vi "IV.vi"(2 "Run uninterrupted?":bool, 3 "Device Category:":string(combo)="Short Strip", 4 "Batch No.:":string, 5 "Wafer Serial No.:":string, 6 "Sensor Serial No.:":string) -> (0 "Done!":bool)   [LabVIEW 2013]
doc: "Performs IV measurements according to ATLAS ITk Quality Control Specifications."
uses:
  InstrControl/Switching/Switching.lvclass
  InstrControl/SupplyControl/SupplyControl.lvclass
  general_VIs/globals/MeasurementSetup.vi
  general_VIs/globals/RunInformation.vi
  InstrControl/InstrumentSetup.vi
  InstrControl/ArduinoControl/ArduinoControl.lvclass
  <vilib>/Analysis/NI_AALBase.lvlib
  InstrControl/InstrControl.lvclass
panel:
  out "Initial volts [V]":dbl format="%.1f"
  out "Final volts [V]":dbl=-700.0 format="%.1f"
  out "step [V]":dbl=10.0 format="%.1f"
  out "step interval [s]":u32=10
  out "Volts":dbl[](array[numeric]) caption="Volts [V]"
  out "Current":dbl[](array[numeric]) caption="Current [nA]"
  out "Temp.":dbl[](array[numeric]) caption="Temp. [°C]" format="%#.2f"
  out "RH":dbl[](array[numeric]) caption="RH [%]" format="%#.2f"
  out "Igraph":cluster{"Initial volts":dbl, dbl, dbl[]}(graph)
  in  "Scales":T1(ring)
  in  "Iscale":enum16{"nanoAmps", "microAmps", "milliAmps"}(ring)
  out "positive ramp?":bool
  out "Tab Control":enum32{"IV Setup", "IV Scan"}(tab)
  in  "User:":string(combo)="Christoph"
  out "IV Supply":string
  in  "Configurations":bool
  in  "Set current limit?":bool
  in  "Current Limit [µA]":dbl=1000.0 min=0.0001 format="%.3f"
  in  "Manufacturer:":string(combo)="Hamamatsu"
  in  "Quit":bool
  in  "Continue":bool
  out "Temperature":enum16{"Read Arduino", "Enter manually"}(ring)
  in  "abort":bool
  out "Device Category:":string
  out "Batch:":string
  out "Current Volts:":dbl format="%.2f"
  in  "quit (no save)":bool
  in  "Quit & Save":bool
  out "Bias On/Off:":bool
  out "STATUS 1":string
  out "Initiated:":string
  out "Sensor No.:":string
  out "No of steps":u32
  out "Current reading No.":u32
  out "Last reading at:":string
  # "University of\nCambridge"
  # "Strip Sensor QC: IV"
  # "IV Scan parameters:"
  # "Last 5 readings:"
  # "n-4"
  # "n-3"
  # "n-2"
  # "n-1"
  # "n"
  # "Vertical Scale:"
  # "DUT & Test Description"
  # "Hardware"
  # "DUT & Test Description:"
  # "Current status:"
  # "Rdg No:"
  # "out of"
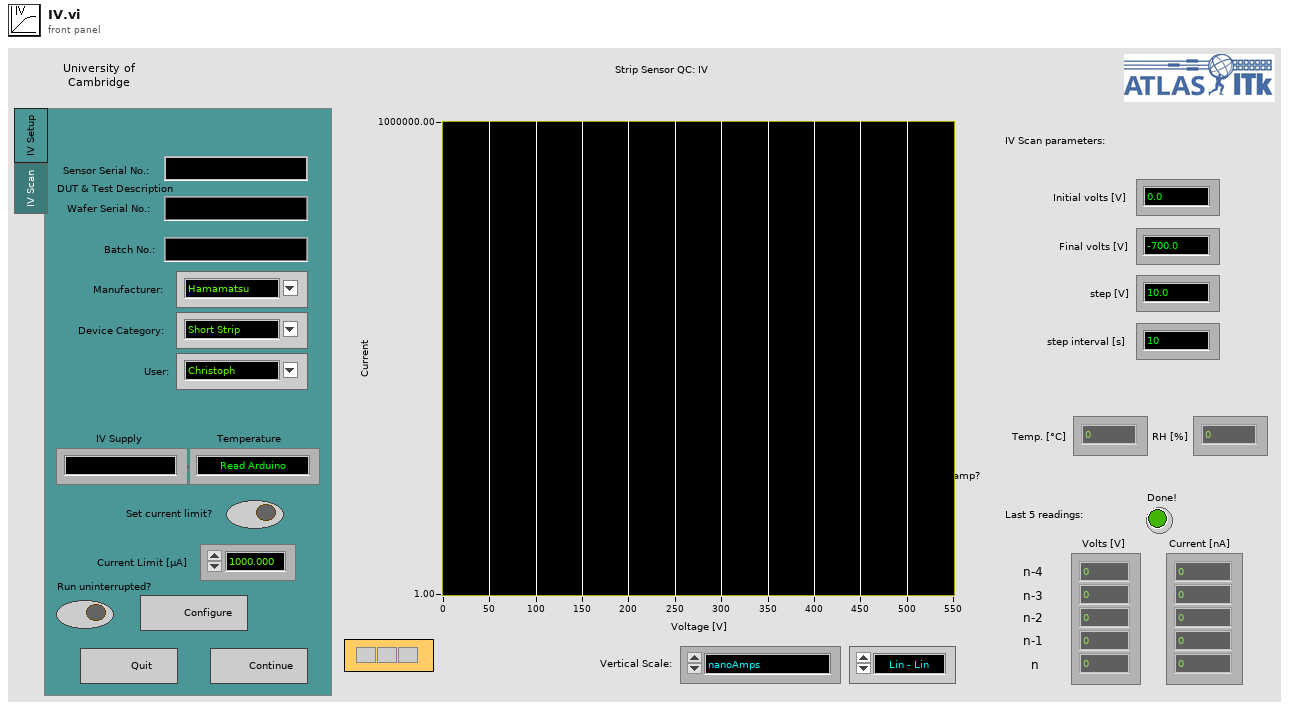
[diagram p1: front panel]
types:
  T1 = enum16{"Lin - Lin", "Log - Lin", "Lin - Log", "Log - log"}
  T2 = enum32{"IV", "CV", "Stability", "Striptest", "Cis", "Ris", "PTP"}
  T3 = enum16{"Reset", "Read Array", "Read Element", "Write Element", "Write Array", "Add Element", "Add Array"}
  T4 = enum16{"Reset", "Ground", "Striptest SMU", "Striptest LCR", "IV", "CV", "Interstrip Cap", "Interstrip Res"}
  T5 = cluster{"Sensor Serial No.:":string, "Wafer Serial No.:":string, "Batch:":string, "Manufacturer:":string, "Device Category:":string, "Database Serial No.:":string, "Initiated:":string, "Test":string, "Instruments used:":string, "Probeplan used:":string, "End of Run comment:":string, "User:":string}
  T6 = cluster{"Institute":string, "Manufacturers":string[], "Devices":string[], "Serialnumbers Lookup DB":string, "Data directory":string, "www directory":string, "List of known users":string[]}
  T7 = cluster{"Supply":refnum<class "SupplyControl.lvclass">, "Initial Voltage [V]":dbl, "Final Voltage [V]":dbl, "Step Size [V]":dbl, "Step Interval [s]":i32, "Number Of Steps":u32, "Ramp down steps [V]":dbl, "Ramp down Interval [s]":i32, "Set Current Limit?":bool, "Current Limit [µA]":dbl, "Temperature Readout":enum16{"Read Arduino", "Enter manually"}, "Arduino":refnum<class "ArduinoControl.lvclass">, "Supply Name":string, "V_breakdown Limit [V]":dbl}
  T8 = cluster{"VISA address":refnum<visa-resource-name>, "T sensor":enum16{"SHT", "DS"}, "Arduino":refnum<class "ArduinoControl.lvclass">}
  T9 = cluster{"GPIB address":string, "Matrix address":string, "Mux1 address":string, "Mux2 address":string, "Matrix used?":bool, "Switching":refnum<class "Switching.lvclass">}
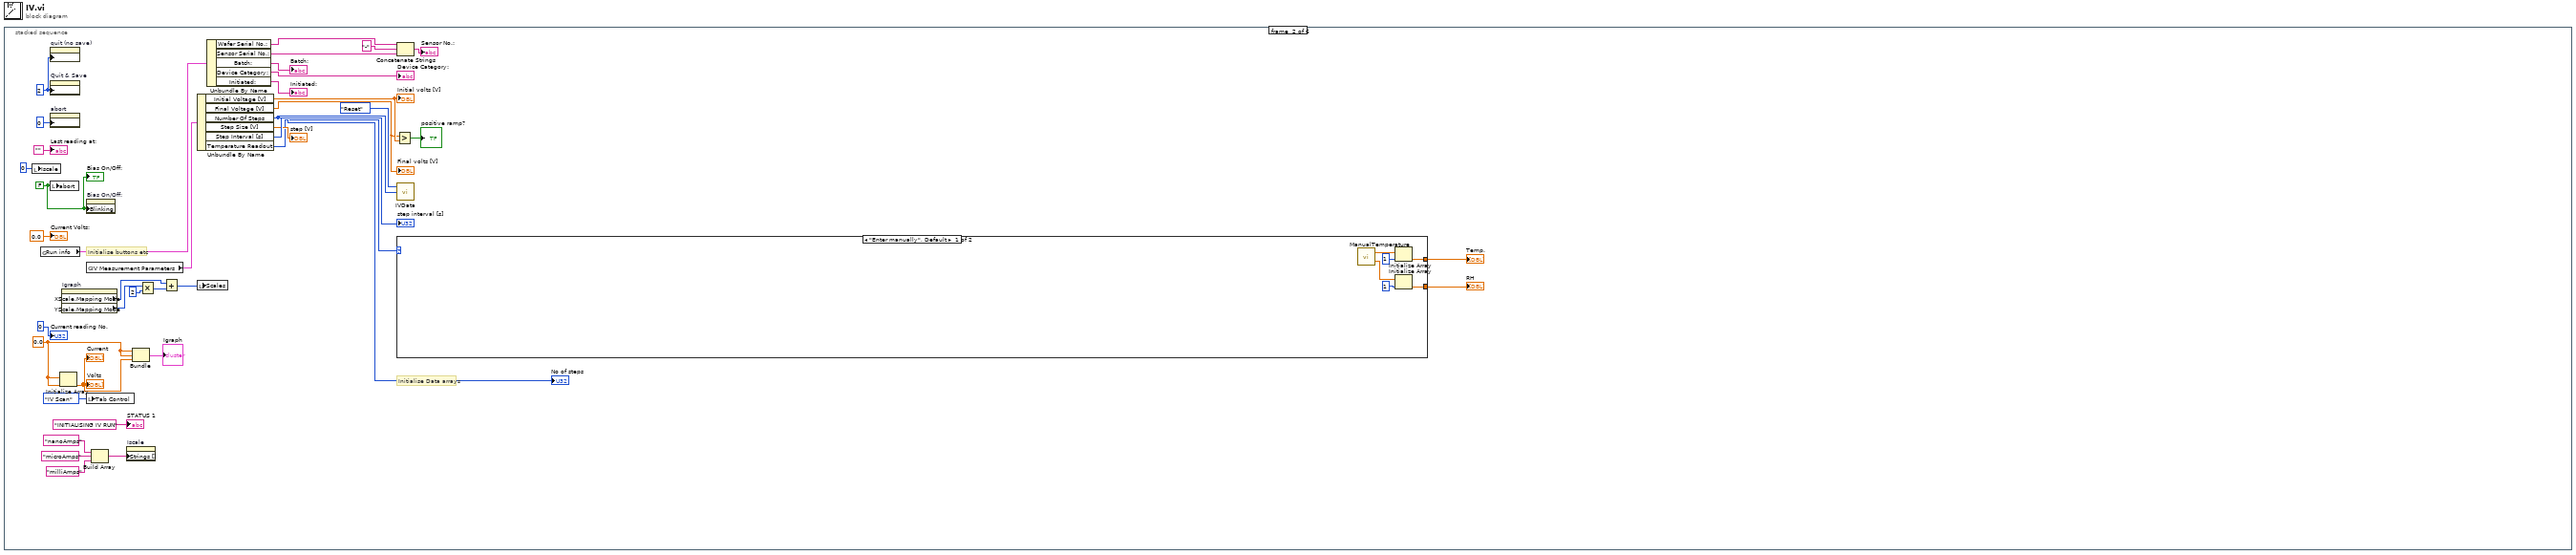
[diagram p0: block diagram]
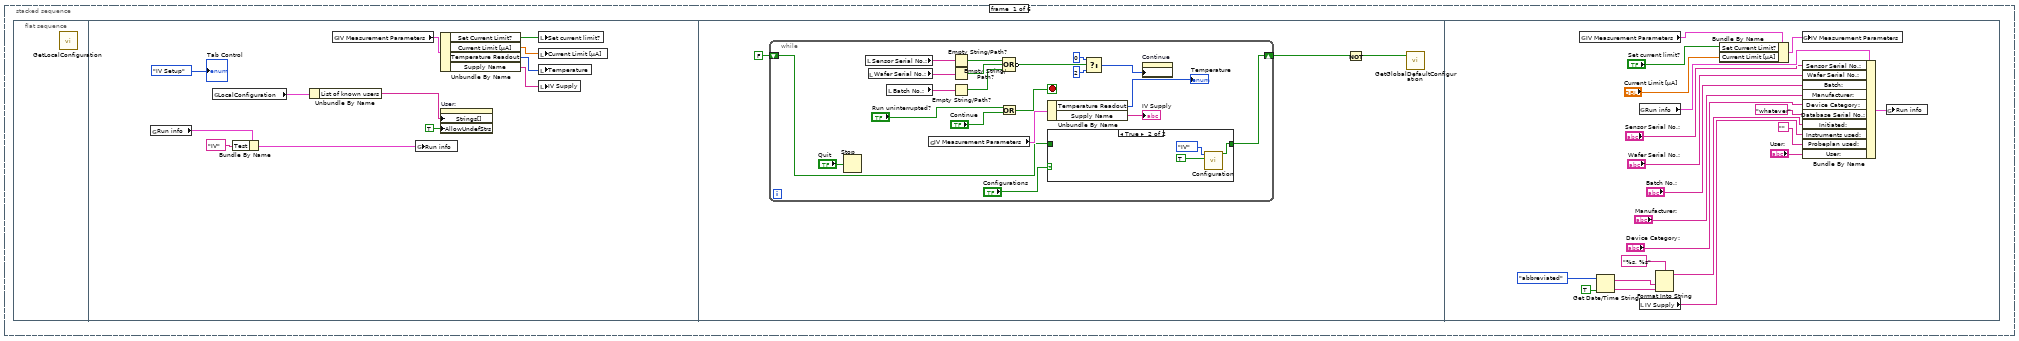
[diagram p2: hidden frame]
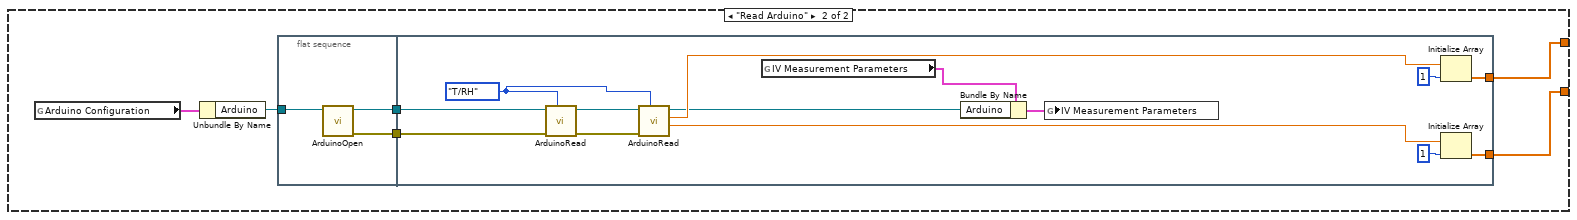
[diagram p4: hidden frame]
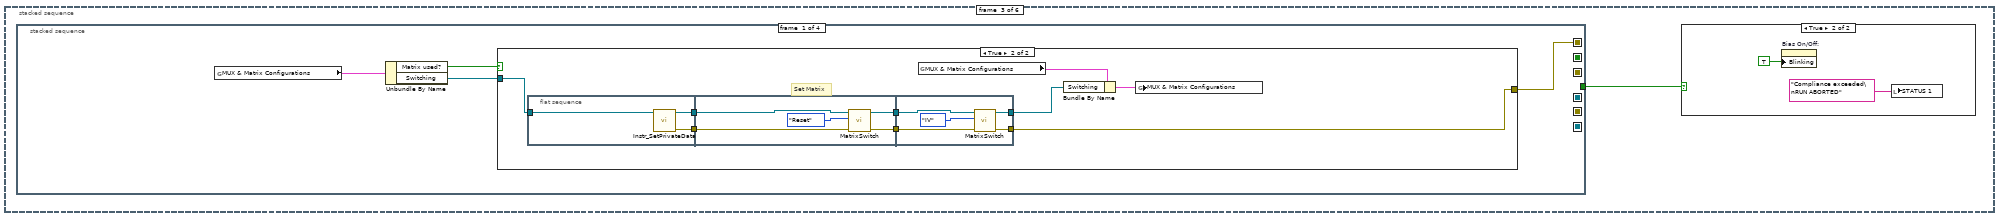
[diagram p5: hidden frame]
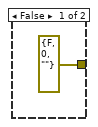
[diagram p6: hidden frame]
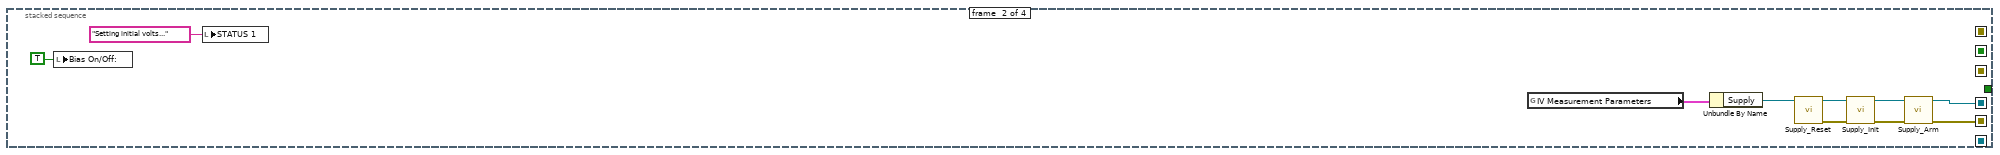
[diagram p7: hidden frame]
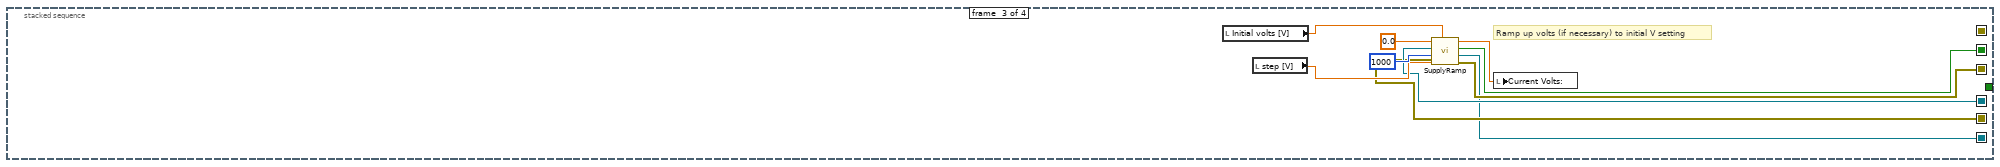
[diagram p8: hidden frame]
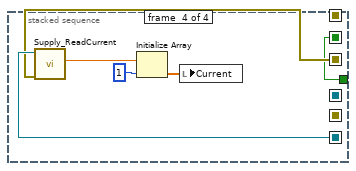
[diagram p9: hidden frame]
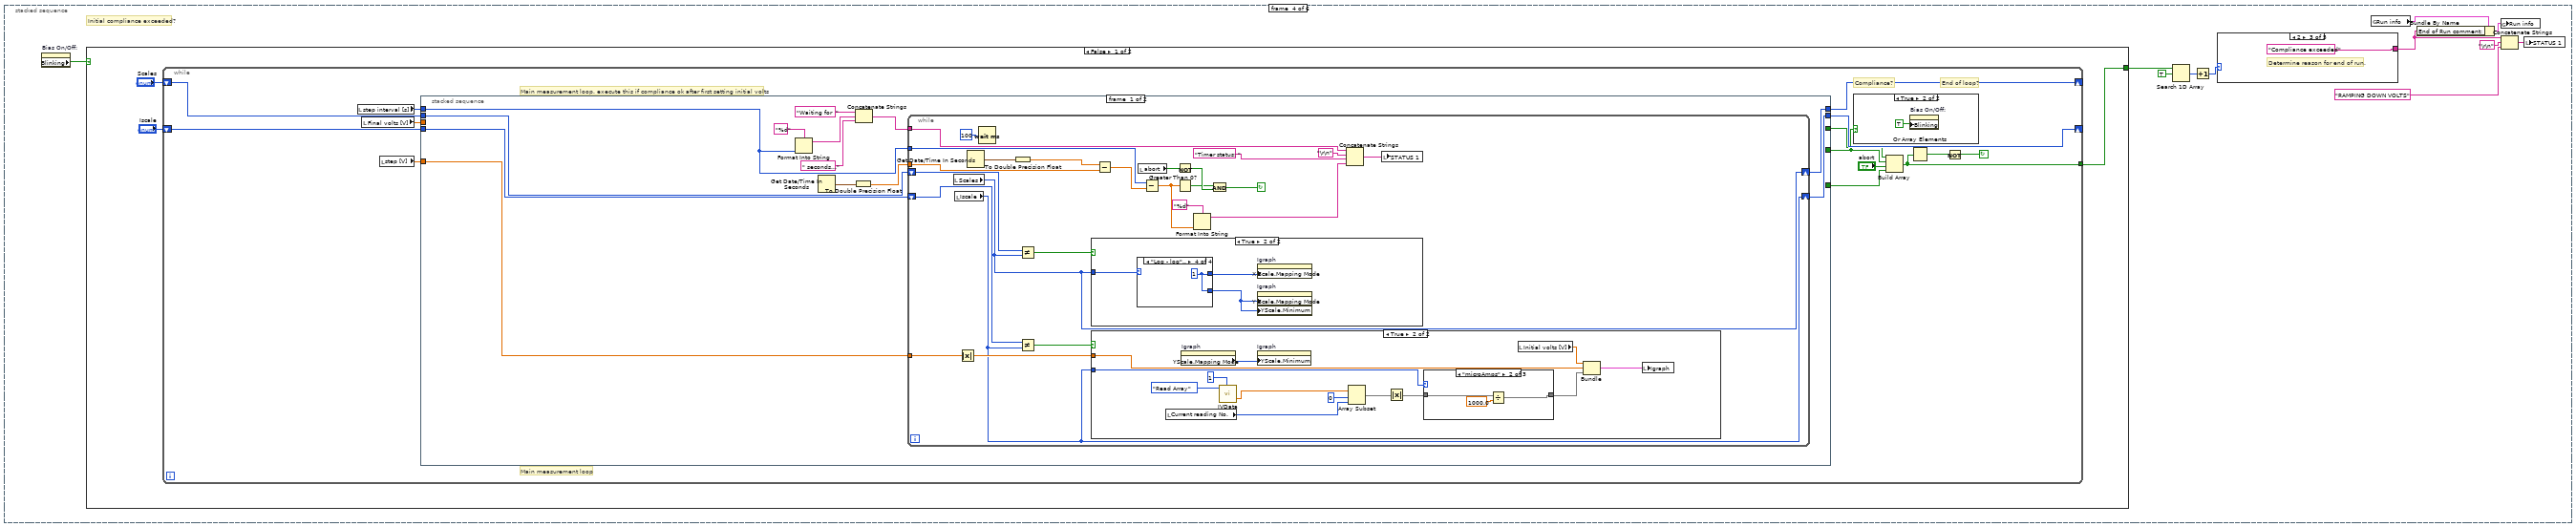
[diagram p11: hidden frame]
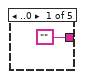
[diagram p12: hidden frame]
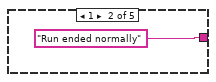
[diagram p13: hidden frame]
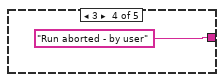
[diagram p14: hidden frame]
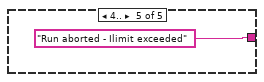
[diagram p15: hidden frame]
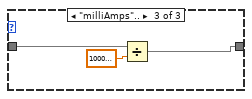
[diagram p18: hidden frame]
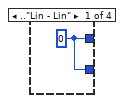
[diagram p20: hidden frame]
diagram:
  n1 = stacked-sequence {
    frame #0 {
      n2 = flat-sequence {
        frame #0 {
          n3 = call "GetLocalConfiguration.vi"() -> ()  [unwired: 3 in, 1 out]
        }
        frame #1 {
          n4 = global read "RunInformation.vi" "Run info"() -> (w3:T5)
          n5 = global read "RunInformation.vi" "LocalConfiguration"() -> (w6:T6)
          n6 = Bundle By Name(cluster=w3, "Test"="IV") -> (w2:T5)
          n7 = Unbundle By Name(w6) -> ("List of known users"=w5:string[])
          n8 = global read "MeasurementSetup.vi" "IV Measurement Parameters"() -> (w9:T7)
          n9 = global write "RunInformation.vi" "Run info"(w2) -> ()
          n10 = Unbundle By Name(w9) -> ("Set Current Limit?"=w8:bool, "Current Limit [µA]"=w7:dbl, "Temperature Readout"=w11:enum16{"Read Arduino", "Enter manually"}, "Supply Name"=w10:string)
          n11 = property on="User:" class="CmbBox"("Strings[]"=w5, "AllowUndefStrs"=TRUE) -> ()  [unwired: 2 in, 2 out]
          n12 = local write "Set current limit?"(w8) -> ()
          n13 = local write "Current Limit [µA]"(w7) -> ()
          n14 = local write "Temperature"(w11) -> ()
          n15 = local write "IV Supply"(w10) -> ()
          "Tab Control" <- enum32{"IV Setup", "IV Scan"}."IV Setup" ("Tab Control")
        }
        frame #2 {
          n16 = while {
            shift-right: [w20] -> w13
            shift-left: FALSE -> [w19]
            stop <- w16 stop-if-true
            n17 = Stop(stop? (T)="Quit") -> ()
            n18 = local read "Sensor Serial No.:"() -> (w34:string)
            n19 = local read "Wafer Serial No.:"() -> (w33:string)
            n20 = local read "Batch No.:"() -> (w25:string)
            n21 = global read "MeasurementSetup.vi" "IV Measurement Parameters"() -> (w23:T7)
            n22 = Empty String/Path?(string/path=w34) -> (empty?=w31:bool)
            n23 = Empty String/Path?(string/path=w33) -> (empty?=w32:bool)
            n24 = Empty String/Path?(string/path=w25) -> (empty?=w24:bool)
            n25 = Or(x="Run uninterrupted?", y="Continue") -> (x .or. y?=w16:bool)
            n26 = Compound Arithmetic op=OR(w31, w32, w24) -> (invert w30:bool)
            n27 = Unbundle By Name(w23) -> ("Temperature Readout"=→"Temperature":enum16{"Read Arduino", "Enter manually"}, "Supply Name"=→"IV Supply":string)
            n28 = case shown="True" "Configurations" {
              tunnel: [w36 w37] -> w20
              tunnel: w19 -> [w36 _]
              frame False {
              }
              frame True {
                n29 = call "Configuration.vi"("Open from\nscan VI"=TRUE, "Measurements"=T2."IV") -> ("configured?"=w37:bool)  [unwired: 9 in]
              }
            }
            n30 = Select(t=0, s=w30, f=2) -> (s? t:f=w27:i32)
            n31 = property on="Continue" class="Bool"("DisabledEnum"=w27) -> ()  [unwired: 2 in, 2 out]
          }
          n32 = Not(x=w13) -> (.not. x?=w14:bool)
          n33 = call "GetGlobalDefaultConfiguration.vi"("Read defaults?"=w14) -> ()  [unwired: 2 in, 1 out]
        }
        frame #3 {
          n34 = global read "MeasurementSetup.vi" "IV Measurement Parameters"() -> (w59:T7)
          n35 = Get Date/Time String(date format (0)=enum16{"short", "long", "abbreviated"}."abbreviated", want seconds? (F)=TRUE) -> (date string=w54:string, time string=w53:string)  [unwired: 1 in]
          n36 = global read "RunInformation.vi" "Run info"() -> (w51:T5)
          n37 = local read "IV Supply"() -> (w43:string)
          n38 = Format Into String(format string="%s, %s", w54, w53) -> (resulting string=w49:string)  [unwired: 2 in, 1 out]
          n39 = Bundle By Name(cluster=w59, "Set Current Limit?"="Set current limit?", "Current Limit [µA]"="Current Limit [µA]") -> (w60:T7)
          n40 = global write "MeasurementSetup.vi" "IV Measurement Parameters"(w60) -> ()
          n41 = Bundle By Name(cluster=w51, "Sensor Serial No.:"="Sensor Serial No.:", "Wafer Serial No.:"="Wafer Serial No.:", "Batch:"="Batch No.:", "Manufacturer:"="Manufacturer:", "Device Category:"="Device Category:", "Database Serial No.:"="whatever", "Initiated:"=w49, "Instruments used:"=w43, "Probeplan used:"="", "User:"="User:") -> (w50:T5)
          n42 = global write "RunInformation.vi" "Run info"(w50) -> ()
        }
      }
    }
    frame #1 {
      w81 = 2
      w89 = 0.0
      w80 = FALSE ("Visible")
      # "Initialise buttons etc"
      # "Initialise Data arrays"
      n43 = local write "Iscale"(u16 0 ("Scale")) -> ()
      n44 = global read "RunInformation.vi" "Run info"() -> (w99:T5)
      n45 = property on="quit (no save)" class="Bool"("DisabledEnum"=w81) -> ()  [unwired: 2 in, 2 out]
      n46 = property on="Quit & Save" class="Bool"("DisabledEnum"=w81) -> ()  [unwired: 2 in, 2 out]
      n47 = property on="abort" class="Bool (strict)"("DisabledEnum"=0) -> ()  [unwired: 2 in, 2 out]
      n48 = local write "abort"(w80) -> ()
      n49 = Initialize Array(w89, w89) -> (w84:dbl[])
      "Volts" <- w84
      "Current" <- w84
      n50 = property on="Igraph" class="WFGraph (strict)"() -> ("XScale.Mapping Mode"=w73:u8, "YScale.Mapping Mode"=w72:u8)  [unwired: 2 in, 2 out]
      n51 = property on="Bias On/Off:" class="Bool (strict)"("Blinking"=w80) -> ()  [unwired: 2 in, 2 out]
      n52 = global read "MeasurementSetup.vi" "IV Measurement Parameters"() -> (w69:T7)
      n53 = local write "Tab Control"(enum32{"IV Setup", "IV Scan"}."IV Scan" ("Tab Control")) -> ()
      n54 = Build Array("nanoAmps", "microAmps", "milliAmps") -> (w96:string[])
      n55 = property on="Iscale" class="Enum (strict)"("Strings []"=w96) -> ()  [unwired: 2 in, 2 out]
      n56 = Bundle(w89, w89, w84) -> (→"Igraph":cluster{dbl, dbl, dbl[]})  [unwired: 1 in]
      n57 = Multiply(x=w72, y=2) -> (x*y=w75:i32)
      n58 = Add(x=w73, y=w75) -> (x+y=w71:i32)
      n59 = Unbundle By Name(w69) -> ("Initial Voltage [V]"=w79:dbl, "Final Voltage [V]"=w78:dbl, "Number Of Steps"=w90:u32, "Step Size [V]"=→"step [V]":dbl, "Step Interval [s]"=→"step interval [s]":i32, "Temperature Readout"=w82:enum16{"Read Arduino", "Enter manually"})
      "No of steps" <- w90
      "Initial volts [V]" <- w79
      "Final volts [V]" <- w78
      n60 = local write "Scales"(w71) -> ()
      n61 = Unbundle By Name(w99) -> ("Wafer Serial No.:"=w66:string, "Sensor Serial No.:"=w65:string, "Batch:"=→"Batch:":string, "Device Category:"=→"Device Category:":string, "Initiated:"=→"Initiated:":string)
      n62 = Greater?(x=w78, y=w79) -> (0:→"positive ramp?":bool)
      n63 = Concatenate Strings(w66, "-", w65) -> (→"Sensor No.:":string)
      n64 = call "IVData.vi"("Action"=T3."Reset", "Array Size / Index"=w90) -> ()  [unwired: 3 in, 2 out]
      n65 = case shown="\"Enter manually\", Default" w82 {
        tunnel: [w105 w112] -> w86
        tunnel: [w102 w111] -> w70
        frame "Enter manually", Default {
          n66 = call "ManualTemperature.vi"() -> ("Humidity [%] out"=w101:dbl, "Temperature [°C] out"=w106:dbl)
          n67 = Initialize Array(w106, 1) -> (w105:dbl[])
          n68 = Initialize Array(w101, 1) -> (w102:dbl[])
        }
        frame "Read Arduino" {
          n69 = global read "InstrumentSetup.vi" "Arduino Configuration"() -> (w108:T8)
          n70 = Unbundle By Name(w108) -> ("Arduino"=w107:refnum<class "ArduinoControl.lvclass">)
          n71 = flat-sequence {
            tunnel: [w113] -> w110
            tunnel: [w115] -> w109
            tunnel: w107 -> [w114]
            tunnel: [w129] -> w112
            tunnel: [w126] -> w111
            tunnel: w110 -> [w120]
            tunnel: w109 -> [w119]
            frame #0 {
              n72 = call "ArduinoOpen.vi"("ArduinoControl in"=w114) -> ("error out"=w115:errorcluster, "ArduinoControl out"=w113:refnum<class "ArduinoControl.lvclass">)  [unwired: 9 in]
            }
            frame #1 {
              w116 = enum16{"T/RH", "Interlock", "Edgesense"}."T/RH" ("Arduino function")
              n73 = call "ArduinoRead.vi"("Arduino function"=w116, "error in (no error)"=w119, "ArduinoControl in"=w120) -> ("error out"=w118:errorcluster, "ArduinoControl out"=w117:refnum<class "ArduinoControl.lvclass">)  [unwired: 3 in, 4 out]
              n74 = call "ArduinoRead.vi"("Arduino function"=w116, "error in (no error)"=w118, "ArduinoControl in"=w117) -> ("rel. Humidity [%]"=w124:dbl, "Temperature [°C]"=w125:dbl, "ArduinoControl out"=w123:refnum<class "ArduinoControl.lvclass">)  [unwired: 3 in, 3 out]
              n75 = global read "MeasurementSetup.vi" "IV Measurement Parameters"() -> (w122:T7)
              n76 = Bundle By Name(cluster=w122, "Arduino"=w123) -> (w121:T7)
              n77 = global write "MeasurementSetup.vi" "IV Measurement Parameters"(w121) -> ()
              n78 = Initialize Array(w125, 1) -> (w129:dbl[])
              n79 = Initialize Array(w124, 1) -> (w126:dbl[])
            }
          }
        }
      }
      "Temp." <- w86
      "RH" <- w70
      "STATUS 1" <- "INITIALISING IV RUN"
      "Bias On/Off:" <- w80
      "Last reading at:" <- ""
      "Current reading No." <- u32 0 ("Current reading No.")
      "Current Volts:" <- 0.0 ("Current Volts:")
    }
    frame #2 {
      n80 = stacked-sequence {
        seq-local: [_ w163 _ _] -> [_ _ w172 _]
        seq-local: [_ w162 _ _] -> [_ _ w171 _]
        seq-local: [_ _ w173 _] -> [_ _ _ w181]
        seq-local: [_ _ w170 _] -> [_ _ _ w182]
        seq-local: [_ _ w169 _] -> [_ _ _ w183]
        seq-local: [w131 _ _ _] -> [_ _ _ _]
        tunnel: [_ _ _ w181] -> w130
        frame #0 {
          n81 = global read "InstrumentSetup.vi" "MUX & Matrix Configurations"() -> (w133:T9)
          n82 = Unbundle By Name(w133) -> ("Matrix used?"=w134:bool, "Switching"=w132:refnum<class "Switching.lvclass">)
          n83 = case shown="True" w134 {
            tunnel: w132 -> [_ w142]
            tunnel: [errorcluster {"status"=FALSE, "code"=0, "source"=""} ("error constant") w136] -> w131
            frame False {
            }
            frame True {
              # "Set Matrix"
              n84 = flat-sequence {
                tunnel: w142 -> [w147]
                tunnel: [w146] -> w141
                tunnel: [w145] -> w140
                tunnel: [w152] -> w144
                tunnel: [w151] -> w143
                tunnel: w141 -> [w150]
                tunnel: w140 -> [w149]
                tunnel: w144 -> [w157]
                tunnel: w143 -> [w156]
                tunnel: [w155] -> w137
                tunnel: [w154] -> w136
                frame #0 {
                  n85 = call-dynamic "Instr_SetPrivateData.vi"("Switching in"=w147) -> ("error out"=w145:errorcluster, "Switching out"=w146:refnum<class "Switching.lvclass">)  [unwired: 9 in]
                }
                frame #1 {
                  n86 = call "MatrixSwitch.vi"("error in (no error)"=w149, "Action"=T4."Reset", "Switching in"=w150) -> ("error out"=w152:errorcluster, "Switching out"=w151:refnum<class "Switching.lvclass">)  [unwired: 7 in]
                }
                frame #2 {
                  n87 = call "MatrixSwitch.vi"("error in (no error)"=w157, "Action"=T4."IV", "Switching in"=w156) -> ("error out"=w154:errorcluster, "Switching out"=w155:refnum<class "Switching.lvclass">)  [unwired: 7 in]
                }
              }
              n88 = global read "InstrumentSetup.vi" "MUX & Matrix Configurations"() -> (w138:T9)
              n89 = Bundle By Name(cluster=w138, "Switching"=w137) -> (w139:T9)
              n90 = global write "InstrumentSetup.vi" "MUX & Matrix Configurations"(w139) -> ()
            }
          }
        }
        frame #1 {
          n91 = local write "Bias On/Off:"(TRUE ("Compliance?")) -> ()
          n92 = local write "STATUS 1"("Setting initial volts..." ("STATUS 1")) -> ()
          n93 = global read "MeasurementSetup.vi" "IV Measurement Parameters"() -> (w161:T7)
          n94 = Unbundle By Name(w161) -> ("Supply"=w158:refnum<class "SupplyControl.lvclass">)
          n95 = call-dynamic "Supply_Reset.vi"("SupplyControl in"=w158) -> ("error out"=w165:errorcluster, "SupplyControl out"=w167:refnum<class "SupplyControl.lvclass">)  [unwired: 9 in]
          n96 = call-dynamic "Supply_Init.vi"("error in (no error)"=w165, "SupplyControl in"=w167) -> ("error out"=w164:errorcluster, "SupplyControl out"=w166:refnum<class "SupplyControl.lvclass">)  [unwired: 8 in]
          n97 = call-dynamic "Supply_Arm.vi"("error in (no error)"=w164, "SupplyControl in"=w166) -> ("error out"=w162:errorcluster, "SupplyControl out"=w163:refnum<class "SupplyControl.lvclass">)  [unwired: 8 in]
        }
        frame #2 {
          # "Ramp up volts (if necessary) to initial V setting"
          n98 = local read "Initial volts [V]"() -> (w168:dbl)
          n99 = local read "step [V]"() -> (w174:dbl)
          n100 = call "SupplyRamp.vi"("error in"=w171, "Requested Voltage"=w168, "Step Size"=w174, "Step Delay"=1000, "Supply IN"=w172, "Starting Voltage"=0.0) -> ("error out"=w170:errorcluster, "Supply OUT"=w169:refnum<class "SupplyControl.lvclass">, "Compliance exceeded"=w173:bool, "Current Voltage"=w177:dbl)  [unwired: 2 in]
          n101 = local write "Current Volts:"(w177) -> ()
        }
        frame #3 {
          n102 = call-dynamic "Supply_ReadCurrent.vi"("error in (no error)"=w182, "SupplyControl in"=w183) -> ("Current in nA"=w179:dbl)  [unwired: 7 in, 2 out]
          n103 = Initialize Array(w179, 1) -> (w178:dbl[])
          n104 = local write "Current"(w178) -> ()
        }
      }
      n105 = case shown="True" w130 {
        frame False {
        }
        frame True {
          n106 = property on="Bias On/Off:" class="Bool (strict)"("Blinking"=TRUE) -> ()  [unwired: 2 in, 2 out]
          n107 = local write "STATUS 1"("Compliance exceeded\nRUN ABORTED") -> ()
        }
      }
    }
    frame #3 {
      # "Initial compliance exceeded?"
      n108 = property on="Bias On/Off:" class="Bool (strict)"() -> ("Blinking"=w196:bool)  [unwired: 2 in, 2 out]
      n109 = case shown="False" w196 {
        tunnel: [w204 w435] -> w195
        frame False {
          n110 = while {
            shift-left: "Iscale" -> [w214]
            shift-right: [w213] -> _
            shift-left: "Scales" -> [w215]
            shift-right: [w216] -> _
            tunnel: [w212] -> w204
            stop <- w217 continue-if-true
            # "Main measurement loop"
            # "End of loop?"
            # "Compliance?"
            # "Main measurement loop. execute this if compliance ok after first setting initial volts"
            n111 = local read "step interval [s]"() -> (w209:u32)
            n112 = local read "Final volts [V]"() -> (w210:dbl)
            n113 = local read "step [V]"() -> (w211:dbl)
            n114 = stacked-sequence {
              tunnel: [w231 _] -> w216
              tunnel: w211 -> [w228 w292]
              tunnel: [_ w291] -> w206
              tunnel: w210 -> [_ w290]
              tunnel: w209 -> [w219 w289]
              tunnel: [_ w288] -> w208
              tunnel: w215 -> [w230 _]
              tunnel: w214 -> [w229 _]
              tunnel: [w227 _] -> w213
              tunnel: [_ w286] -> w207
              frame #0 {
                n115 = Format Into String(format string="%d", w219) -> (resulting string=w224:string)  [unwired: 2 in, 1 out]
                n116 = Get Date/Time In Seconds() -> (seconds since 1Jan1904=w221:timestamp)
                n117 = To Double Precision Float(number=w221) -> (double precision float=w222:dbl)
                n118 = Concatenate Strings("Waiting for  ", w224, " seconds...") -> (w220:string)
                n119 = while {
                  tunnel: w228 -> [w240]
                  shift-left: w229 -> [w244]
                  shift-right: [w237] -> w227
                  shift-left: w230 -> [w245]
                  shift-right: [w246] -> w231
                  tunnel: w220 -> [w238]
                  tunnel: w219 -> [w250]
                  tunnel: w222 -> [w251]
                  stop <- w252 continue-if-true
                  n120 = local read "Scales"() -> (w246:T1)
                  n121 = local read "Iscale"() -> (w237:enum16{"nanoAmps", "microAmps", "milliAmps"})
                  n122 = Absolute Value(x=w240) -> (abs(x)=w239:dbl)
                  n123 = Get Date/Time In Seconds() -> (seconds since 1Jan1904=w236:timestamp)
                  n124 = Wait (ms)(milliseconds to wait=u32 100) -> ()  [unwired: 1 out]
                  n125 = To Double Precision Float(number=w236) -> (double precision float=w256:dbl)
                  n126 = Not Equal?(x=w245, y=w246) -> (x != y?=w247:bool)
                  n127 = Not Equal?(x=w244, y=w237) -> (x != y?=w235:bool)
                  n128 = case shown="True" w247 {
                    tunnel: w246 -> [_ w279]
                    frame False {
                    }
                    frame True {
                      n129 = case shown="\"Log - log\".." w279 {
                        tunnel: [w280 1 0 w285] -> w278
                        tunnel: [w280 0 1 w285] -> w277
                        frame .."Lin - Lin" {
                          w280 = 0
                        }
                        frame "Log - Lin" {
                        }
                        frame "Lin - Log" {
                        }
                        frame "Log - log".. {
                          w285 = 1
                        }
                      }
                      n130 = property on="Igraph" class="WFGraph (strict)"("X Scale.Mapping Mode"=w278) -> ()  [unwired: 2 in, 2 out]
                      n131 = property on="Igraph" class="WFGraph (strict)"("Y Scale.Mapping Mode"=w277, "YScale.Minimum"=w277) -> ()  [unwired: 2 in, 2 out]
                    }
                  }
                  n132 = case shown="True" w235 {
                    tunnel: w239 -> [_ w266]
                    tunnel: w237 -> [_ w262]
                    frame False {
                    }
                    frame True {
                      n133 = local read "Current reading No."() -> (w264:u32)
                      n134 = property on="Igraph" class="WFGraph (strict)"() -> ("YScale.Mapping Mode"=w258:u8)  [unwired: 2 in, 2 out]
                      n135 = call "IVData.vi"("Action"=T3."Read Array", "Array No."=u32 1 ("Action")) -> ("Array OUT"=w267:dbl[])  [unwired: 3 in, 1 out]
                      n136 = property on="Igraph" class="WFGraph (strict)"("YScale.Minimum"=w258) -> ()  [unwired: 2 in, 2 out]
                      n137 = Array Subset(array=w267, index=0, length=w264) -> (w261:dbl[])
                      n138 = Absolute Value(x=w261) -> (abs(x)=w260:dbl[])
                      n139 = case shown="\"microAmps\"" w262 {
                        tunnel: [w270 w271 w275] -> w269
                        tunnel: w260 -> [w270 w273 w276]
                        frame .."nanoAmps" {
                        }
                        frame "microAmps" {
                          n140 = Divide(x=w273, y=1000.0) -> (x/y=w271:dbl[])
                        }
                        frame "milliAmps".. {
                          n141 = Divide(x=w276, y=1000000.0) -> (x/y=w275:dbl[])
                        }
                      }
                      n142 = local read "Initial volts [V]"() -> (w265:dbl)
                      n143 = Bundle("Initial volts [V]"=w265, w266, w269) -> (w263:cluster{"Initial volts [V]":dbl, dbl, dbl[]})  [unwired: 1 in]
                      n144 = local write "Igraph"(w263) -> ()
                    }
                  }
                  n145 = Subtract(x=w256, y=w251) -> (x-y=w233:dbl)
                  n146 = local read "abort"() -> (w249:bool)
                  n147 = Subtract(x=w250, y=w233) -> (x-y=w232:dbl)
                  n148 = Not(x=w249) -> (.not. x?=w255:bool)
                  n149 = Greater Than 0?(x=w232) -> (x > 0?=w234:bool)
                  n150 = Format Into String(format string="%d", w232) -> (resulting string=w254:string)  [unwired: 2 in, 1 out]
                  n151 = And(x=w234, y=w255) -> (x .and. y?=w252:bool)
                  n152 = Concatenate Strings(w238, "\r\n", "Timer status: ", w254) -> (w248:string)
                  n153 = local write "STATUS 1"(w248) -> ()
                }
              }
              frame #1 {
                n154 = local read "abort"() -> (w287:bool)
                n155 = case shown="False" w287 {
                  tunnel: [w298 w432] -> w288
                  tunnel: w289 -> [w297 _]
                  tunnel: w290 -> [w296 _]
                  tunnel: [w294 w432] -> w291
                  tunnel: w292 -> [w295 _]
                  tunnel: [w293 w432] -> w286
                  frame False {
                    n156 = stacked-sequence {
                      seq-local: [w313 _ _] -> [_ w339 _]
                      seq-local: [w308 _ _] -> [_ _ w401]
                      seq-local: [w307 _ _] -> [_ _ w402]
                      tunnel: w295 -> [_ w353 w407]
                      tunnel: w296 -> [_ _ w398]
                      tunnel: [_ _ w405] -> w298
                      tunnel: [_ _ w404] -> w294
                      tunnel: w297 -> [_ _ _]
                      tunnel: [w317 _ _] -> w293
                      frame #0 {
                        w311 = T3."Write Element" ("Action")
                        # "SMU data"
                        n157 = Get Date/Time String(want seconds? (F)=TRUE) -> (time string=w314:string)  [unwired: 2 in, 1 out]
                        n158 = local write "Last reading at:"(w314) -> ()
                        n159 = local write "STATUS 1"("Reading current ..." ("status")) -> ()
                        n160 = global read "MeasurementSetup.vi" "IV Measurement Parameters"() -> (w306:T7)
                        n161 = Unbundle By Name(w306) -> ("Supply"=w300:refnum<class "SupplyControl.lvclass">, "Set Current Limit?"=w305:bool, "Current Limit [µA]"=w302:dbl, "Temperature Readout"=w304:enum16{"Read Arduino", "Enter manually"}, "Arduino"=w299:refnum<class "ArduinoControl.lvclass">)
                        n162 = case shown="\"Read Arduino\"" w304 {
                          tunnel: [w327 w333] -> w315
                          tunnel: [w324 w332] -> w309
                          tunnel: w299 -> [_ w331]
                          frame "Enter manually", Default {
                            n163 = local read "Temp."() -> (w329:dbl[])
                            n164 = local read "RH"() -> (w325:dbl[])
                            n165 = Index Array(array=w325, index=0) -> (element=w324:dbl)
                            n166 = Index Array(array=w329, index=0) -> (element=w327:dbl)
                          }
                          frame "Read Arduino" {
                            n167 = call "ArduinoRead.vi"("Arduino function"=enum16{"T/RH", "Interlock", "Edgesense"}."T/RH", "ArduinoControl in"=w331) -> ("rel. Humidity [%]"=w332:dbl, "Temperature [°C]"=w333:dbl)  [unwired: 4 in, 4 out]
                          }
                        }
                        n168 = Multiply(x=w302, y=1000.0) -> (x*y=w301:dbl)
                        n169 = local read "Current reading No."() -> (w310:u32)
                        n170 = call-dynamic "Supply_ReadCurrent.vi"("SupplyControl in"=w300) -> ("error out"=w307:errorcluster, "Current in nA"=w318:dbl, "SupplyControl out"=w308:refnum<class "SupplyControl.lvclass">)  [unwired: 8 in]
                        n171 = local read "Current Volts:"() -> (w319:dbl)
                        n172 = case shown="True" w305 {
                          tunnel: w318 -> [_ w338]
                          tunnel: w301 -> [_ w336]
                          tunnel: [FALSE w335] -> w317
                          frame False {
                          }
                          frame True {
                            n173 = Absolute Value(x=w338) -> (abs(x)=w337:dbl)
                            n174 = Greater?(x=w337, y=w336) -> (0:w335:bool)
                          }
                        }
                        n175 = Increment(x=w310) -> (x+1=w313:u32)
                        n176 = call "IVData.vi"("Action"=w311, "Array No."=u32 1, "Array Size / Index"=w310, "Data IN"=w318) -> ()  [unwired: 1 in, 2 out]
                        n177 = call "IVData.vi"("Action"=w311, "Array No."=0, "Array Size / Index"=w310, "Data IN"=w319) -> ()  [unwired: 1 in, 2 out]
                        n178 = local write "Current reading No."(w313) -> ()
                        n179 = call "IVData.vi"("Action"=w311, "Array No."=u32 2, "Array Size / Index"=w310, "Data IN"=w315) -> ()  [unwired: 1 in, 2 out]
                        n180 = call "IVData.vi"("Action"=w311, "Array No."=u32 3, "Array Size / Index"=w310, "Data IN"=w309) -> ()  [unwired: 1 in, 2 out]
                      }
                      frame #1 {
                        w350 = u32 5 ("y")
                        # "Update plots"
                        n181 = property on="Igraph" class="WFGraph (strict)"() -> ("YScale.Mapping Mode"=w341:u8)  [unwired: 2 in, 2 out]
                        n182 = property on="Igraph" class="WFGraph (strict)"("YScale.Minimum"=w341) -> ()  [unwired: 2 in, 2 out]
                        n183 = call "IVData.vi"("Action"=T3."Read Array", "Array No."=1) -> ("Array OUT"=w355:dbl[])  [unwired: 3 in, 1 out]
                        n184 = Greater?(x=w339, y=w350) -> (0:w349:bool)
                        n185 = case shown="True" w349 {
                          tunnel: w339 -> [w359 w362]
                          tunnel: w350 -> [_ w361]
                          tunnel: [w359 w361] -> w348
                          tunnel: [0 w360] -> w346
                          frame False {
                          }
                          frame True {
                            n186 = Subtract(x=w362, y=w361) -> (x-y=w360:u32)
                          }
                        }
                        n187 = Array Subset(array=w355, index=0, length=w339) -> (w345:dbl[])
                        n188 = Absolute Value(x=w345) -> (abs(x)=w344:dbl[])
                        n189 = local read "Iscale"() -> (w351:enum16{"nanoAmps", "microAmps", "milliAmps"})
                        n190 = case shown="\"microAmps\"" w351 {
                          tunnel: [w387 w388 w391] -> w357
                          tunnel: w344 -> [w387 w390 w393]
                          frame .."nanoAmps" {
                          }
                          frame "microAmps" {
                            n191 = Divide(x=w390, y=1000.0) -> (x/y=w388:dbl[])
                          }
                          frame "milliAmps".. {
                            n192 = Divide(x=w393, y=1000000.0) -> (x/y=w391:dbl[])
                          }
                        }
                        n193 = for {
                          N: 4 -> [_]
                          tunnel: w348 -> [w367]
                          tunnel: w346 -> [w366]
                          tunnel: w339 -> [w363]
                          i -> [w368]
                          n194 = call "IVData.vi"("Action"=T3."Read Array", "Array No."=w368) -> ("Array OUT"=w365:dbl[])  [unwired: 3 in, 1 out]
                          n195 = case shown="2" w368 {
                            tunnel: w367 -> [w371 w375 _ _]
                            tunnel: w366 -> [w372 w376 _ _]
                            tunnel: w365 -> [w370 w374 w380 w385]
                            tunnel: w363 -> [_ _ w378 w383]
                            frame ..0 {
                              n196 = Array Subset(array=w370, index=w372, length=w371) -> (w369:dbl[])
                              n197 = local write "Volts"(w369) -> ()
                            }
                            frame 1 {
                              n198 = Array Subset(array=w374, index=w376, length=w375) -> (w373:dbl[])
                              n199 = local write "Current"(w373) -> ()
                            }
                            frame 2 {
                              n200 = Decrement(x=w378) -> (x-1=w377:u32)
                              n201 = Array Subset(array=w380, index=w377, length=1) -> (w379:dbl[])
                              n202 = local write "Temp."(w379) -> ()
                            }
                            frame 3.. {
                              n203 = Decrement(x=w383) -> (x-1=w382:u32)
                              n204 = Array Subset(array=w385, index=w382, length=1) -> (w384:dbl[])
                              n205 = local write "RH"(w384) -> ()
                            }
                          }
                        }
                        n206 = local read "Initial volts [V]"() -> (w354:dbl)
                        n207 = Absolute Value(x=w353) -> (abs(x)=w352:dbl)
                        n208 = Bundle("Initial volts [V]"=w354, w352, w357) -> (w342:cluster{"Initial volts [V]":dbl, dbl, dbl[]})  [unwired: 1 in]
                        n209 = local write "Igraph"(w342) -> ()
                      }
                      frame #2 {
                        # "Increment volts and check for end of loop"
                        n210 = local read "positive ramp?"() -> (w403:bool)
                        n211 = local read "Current Volts:"() -> (w399:dbl)
                        n212 = case shown="True" w403 {
                          tunnel: w398 -> [w410 w414]
                          tunnel: w407 -> [w411 w417]
                          tunnel: [w409 w416] -> w394
                          tunnel: [w408 w413] -> w406
                          tunnel: w399 -> [w412 w415]
                          frame False {
                            n213 = Subtract(x=w412, y=w411) -> (x-y=w408:dbl)
                            n214 = Greater Or Equal?(x=w408, y=w410) -> (x >= y?=w409:bool)
                          }
                          frame True {
                            n215 = Add(x=w415, y=w417) -> (x+y=w413:dbl)
                            n216 = Less Or Equal?(x=w413, y=w414) -> (x <= y?=w416:bool)
                          }
                        }
                        n217 = Quotient & Remainder(x=w399, y=w398) -> (x-y*floor(x/y)=w400:dbl, floor(x/y)=w397:dbl)
                        n218 = Not Equal To 0?(x=w400) -> (x != 0?=w395:bool)
                        n219 = Equal To 0?(x=w397) -> (x = 0?=w396:bool)
                        n220 = Or(x=w395, y=w396) -> ()  [unwired: 1 out]
                        n221 = case shown="True" w394 {
                          tunnel: w406 -> [_ w428]
                          tunnel: [TRUE FALSE] -> w405
                          tunnel: [FALSE w429] -> w404
                          tunnel: w399 -> [_ w426]
                          tunnel: w402 -> [_ w425]
                          tunnel: w401 -> [_ w424]
                          frame False {
                          }
                          frame True {
                            n222 = local read "step [V]"() -> (w422:dbl)
                            n223 = local write "STATUS 1"("Incrementing volts.") -> ()
                            n224 = call "SupplyRamp.vi"("error in"=w425, "Requested Voltage"=w428, "Step Size"=w422, "Step Delay"=100, "Supply IN"=w424, "Starting Voltage"=w426) -> ("error out"=w420:errorcluster, "Compliance exceeded"=w429:bool, "Current Voltage"=w423:dbl)  [unwired: 2 in, 1 out]
                            n225 = case shown="No Error" w420 {
                              tunnel: w423 -> [w431 _]
                              frame No Error {
                                n226 = local write "Current Volts:"(w431) -> ()
                              }
                              frame Error {
                              }
                            }
                            n227 = property on="Bias On/Off:" class="Bool (strict)"("Blinking"=w429) -> ()  [unwired: 2 in, 2 out]
                          }
                        }
                      }
                    }
                  }
                  frame True {
                    w432 = FALSE
                  }
                }
              }
            }
            n228 = case shown="True" w206 {
              frame False {
              }
              frame True {
                n229 = property on="Bias On/Off:" class="Bool (strict)"("Blinking"=TRUE) -> ()  [unwired: 2 in, 2 out]
              }
            }
            n230 = Build Array(w208, w206, "abort", w207) -> (w212:bool[])
            n231 = Or Array Elements(Boolean array=w212) -> (logical OR=w218:bool)
            n232 = Not(x=w218) -> (.not. x?=w217:bool)
          }
        }
        frame True {
          w434 = FALSE
          # "compliance was exceeded when first voltage applied."
          # "Flag compliance as reason for end of run"
          n233 = local write "STATUS 1"("Run aborted - compliance exceeded.") -> ()
          n234 = Build Array(w434, TRUE, w434, w434) -> (w435:bool[])
        }
      }
      n235 = Search 1D Array(1D array=w195, element=TRUE) -> (index of element=w193:i32)  [unwired: 1 in]
      n236 = Increment(x=w193) -> (x+1=w192:i32)
      n237 = case shown="2" w192 {
        tunnel: ["" "Run ended normally" "Compliance exceeded" "Run aborted - by user" "Run aborted - Ilimit exceeded"] -> w187
        frame ..0 {
        }
        frame 1 {
        }
        frame 2 {
          # "Determine reason for end of run."
        }
        frame 3 {
        }
        frame 4.. {
        }
      }
      n238 = global read "RunInformation.vi" "Run info"() -> (w191:T5)
      n239 = Bundle By Name(cluster=w191, "End of Run comment:"=w187) -> (w186:T5)
      n240 = global write "RunInformation.vi" "Run info"(w186) -> ()
      n241 = Concatenate Strings(w187, "\r\n", "RAMPING DOWN VOLTS") -> (w190:string)
      n242 = local write "STATUS 1"(w190) -> ()
    }
    frame #4 {
      n243 = stacked-sequence {
        seq-local: [w440 _ _ _ _] -> [_ w451 _ _ _]
        seq-local: [w439 _ _ _ _] -> [_ w450 _ _ _]
        seq-local: [_ w449 _ _ _] -> [_ _ w452 _ _]
        frame #0 {
          # "Ramp down volts now"
          n244 = global read "MeasurementSetup.vi" "IV Measurement Parameters"() -> (w443:T7)
          n245 = Unbundle By Name(w443) -> ("Supply"=w438:refnum<class "SupplyControl.lvclass">, "Ramp down steps [V]"=w442:dbl, "Ramp down Interval [s]"=w441:i32)
          n246 = Multiply(x=w441, y=1000) -> (x*y=w445:i32)
          n247 = local read "Current Volts:"() -> (w448:dbl)
          n248 = call "SupplyRamp.vi"("Requested Voltage"=0.0, "Step Size"=w442, "Step Delay"=w445, "Supply IN"=w438, "Starting Voltage"=w448) -> ("error out"=w440:errorcluster, "Supply OUT"=w439:refnum<class "SupplyControl.lvclass">, "Current Voltage"=w446:dbl)  [unwired: 3 in, 1 out]
          n249 = local write "Current Volts:"(w446) -> ()
        }
        frame #1 {
          # "Tie up loose ends. Set volts to zero and switch to standby"
          n250 = call-dynamic "Supply_Stby.vi"("error in (no error)"=w451, "SupplyControl in"=w450) -> ("error out"=w449:errorcluster)  [unwired: 8 in, 1 out]
        }
        frame #2 {
          n251 = global read "InstrumentSetup.vi" "MUX & Matrix Configurations"() -> (w454:T9)
          n252 = Unbundle By Name(w454) -> ("Matrix used?"=w455:bool, "Switching"=w453:refnum<class "Switching.lvclass">)
          n253 = case shown="True" w455 {
            tunnel: w453 -> [_ w458]
            tunnel: w452 -> [_ w457]
            frame False {
            }
            frame True {
              n254 = call "MatrixSwitch.vi"("error in (no error)"=w457, "Action"=T4."Reset", "Switching in"=w458) -> ()  [unwired: 7 in, 2 out]
            }
          }
        }
        frame #3 {
          w463 = 0
          n255 = local write "Bias On/Off:"(FALSE ("Visible")) -> ()
          n256 = local write "Current Volts:"(0.0 ("Current Volts:")) -> ()
          n257 = property on="abort" class="Bool (strict)"("DisabledEnum"=2) -> ()  [unwired: 2 in, 2 out]
          n258 = property on="Quit & Save" class="Bool"("DisabledEnum"=w463) -> ()  [unwired: 2 in, 2 out]
          n259 = property on="quit (no save)" class="Bool"("DisabledEnum"=w463) -> ()  [unwired: 2 in, 2 out]
          n260 = local write "STATUS 1"("Run finished. \nSave data?" ("STATUS 1")) -> ()
        }
        frame #4 {
          n261 = Current VI's Path() -> (path=w465:path)
          n262 = call "SaveJPEG.vi"("Test"="IV", "File Path Control"=w465) -> ()  [unwired: 1 in, 2 out]
        }
      }
    }
    frame #5 {
      # "Loop and await decision on whether to save or junk data"
      n263 = local read "Scales"() -> (w476:T1)
      n264 = local read "Iscale"() -> (w475:enum16{"nanoAmps", "microAmps", "milliAmps"})
      n265 = while {
        shift-left: w475 -> [w516]
        shift-right: [w515] -> _
        shift-left: w476 -> [w518]
        shift-right: [w517] -> _
        tunnel: ["Quit & Save"] -> w478
        tunnel: ["quit (no save)"] -> w477
        stop <- w513 continue-if-true
        n266 = local read "Scales"() -> (w517:T1)
        n267 = local read "Iscale"() -> (w515:enum16{"nanoAmps", "microAmps", "milliAmps"})
        n268 = Not Equal?(x=w518, y=w517) -> (x != y?=w511:bool)
        n269 = Not Equal?(x=w516, y=w515) -> (x != y?=w510:bool)
        n270 = case shown="True" w511 {
          tunnel: w517 -> [_ w543]
          frame False {
          }
          frame True {
            n271 = case shown="..\"Lin - Lin\"" w543 {
              tunnel: [w544 1 0 w549] -> w542
              tunnel: [w544 0 1 w549] -> w541
              frame .."Lin - Lin" {
                w544 = 0
              }
              frame "Log - Lin" {
              }
              frame "Lin - Log" {
              }
              frame "Log - log".. {
                w549 = 1
              }
            }
            n272 = property on="Igraph" class="WFGraph (strict)"("X Scale.Mapping Mode"=w542) -> ()  [unwired: 2 in, 2 out]
            n273 = property on="Igraph" class="WFGraph (strict)"("Y Scale.Mapping Mode"=w541, "YScale.Minimum"=w541) -> ()  [unwired: 2 in, 2 out]
          }
        }
        n274 = case shown="True" w510 {
          tunnel: w515 -> [_ w529]
          frame False {
          }
          frame True {
            n275 = property on="Igraph" class="WFGraph (strict)"() -> ("YScale.Mapping Mode"=w521:u8)  [unwired: 2 in, 2 out]
            n276 = property on="Igraph" class="WFGraph (strict)"("YScale.Minimum"=w521) -> ()  [unwired: 2 in, 2 out]
            n277 = global read "MeasurementSetup.vi" "IV Measurement Parameters"() -> (w519:T7)
            n278 = Unbundle By Name(w519) -> ("Initial Voltage [V]"=w523:dbl, "Step Size [V]"=w525:dbl, "Number Of Steps"=w522:u32)
            n279 = call "IVData.vi"("Action"=T3."Read Array", "Array No."=u32 1 ("Action")) -> ("Array OUT"=w531:dbl[])  [unwired: 3 in, 1 out]
            n280 = Absolute Value(x=w525) -> (abs(x)=w524:dbl)
            n281 = Array Subset(array=w531, index=0, length=w522) -> (w528:dbl[])
            n282 = Absolute Value(x=w528) -> (abs(x)=w527:dbl[])
            n283 = case shown="..\"nanoAmps\"" w529 {
              tunnel: [w534 w535 w539] -> w533
              tunnel: w527 -> [w534 w537 w540]
              frame .."nanoAmps" {
              }
              frame "microAmps" {
                n284 = Divide(x=w537, y=1000.0) -> (x/y=w535:dbl[])
              }
              frame "milliAmps".. {
                n285 = Divide(x=w540, y=1000000.0) -> (x/y=w539:dbl[])
              }
            }
            n286 = Bundle("Initial Voltage [V]"=w523, w524, w533) -> (w530:cluster{"Initial Voltage [V]":dbl, dbl, dbl[]})  [unwired: 1 in]
            n287 = local write "Igraph"(w530) -> ()
          }
        }
        n288 = Not Or(1:"quit (no save)", 2:"Quit & Save") -> (0:w513:bool)
      }
      n289 = global read "MeasurementSetup.vi" "IV Measurement Parameters"() -> (w474:T7)
      n290 = Unbundle By Name(w474) -> ("Temperature Readout"=w473:enum16{"Read Arduino", "Enter manually"}, "Arduino"=w467:refnum<class "ArduinoControl.lvclass">)
      n291 = case shown="\"Read Arduino\"" w473 {
        tunnel: w467 -> [_ w509]
        frame "Enter manually", Default {
        }
        frame "Read Arduino" {
          n292 = call "ArduinoClose.vi"("ArduinoControl in"=w509) -> ()  [unwired: 9 in, 2 out]
        }
      }
      n293 = case shown="True" w477 {
        tunnel: [FALSE w551] -> w479
        frame False {
        }
        frame True {
          n294 = Two Button Dialog(message="Are you sure you don't want to save the data?", 1:"Quit" ("F button name (\"Cancel\")"), 2:"Save data" ("T button name (\"OK\")")) -> (T button?=w551:bool)
        }
      }
      n295 = Or(x=w478, y=w479) -> (x .or. y?=w472:bool)
      n296 = flat-sequence {
        tunnel: w472 -> [w489]
        tunnel: [w489] -> w468
        tunnel: [TRUE] -> w466
        frame #0 {
          w501 = T3."Read Array" ("Action")
          n297 = global read "MeasurementSetup.vi" "IV Measurement Parameters"() -> (w504:T7)
          n298 = local write "STATUS 1"("Saving Data ...") -> ()
          n299 = call "IVData.vi"("Action"=w501, "Array No."=u32 0 ("Action")) -> ("Array OUT"=w496:dbl[])  [unwired: 3 in, 1 out]
          n300 = call "IVData.vi"("Action"=w501, "Array No."=u32 1 ("Action")) -> ("Array OUT"=w495:dbl[])  [unwired: 3 in, 1 out]
          n301 = Unbundle By Name(w504) -> ("V_breakdown Limit [V]"=w481:dbl, "Number Of Steps"=w484:u32)
          n302 = Build Array(w496, w495) -> (w494:dbl[][])
          n303 = call "IVData.vi"("Action"=w501, "Array No."=u32 3 ("Action")) -> ("Array OUT"=w503:dbl[])  [unwired: 3 in, 1 out]
          n304 = call "IVData.vi"("Action"=w501, "Array No."=u32 2 ("Action")) -> ("Array OUT"=w502:dbl[])  [unwired: 3 in, 1 out]
          n305 = call "ScanFeedback.vi"("measurement type"=T2."IV") -> ("V breakdown"=w483:dbl)  [unwired: 3 in, 5 out]
          n306 = call <vilib>:"Std Deviation and Variance.vi"("X"=w503) -> ("mean"=w490:dbl)  [unwired: 1 in, 2 out]
          n307 = call <vilib>:"Std Deviation and Variance.vi"("X"=w502) -> ("mean"=w491:dbl)  [unwired: 1 in, 2 out]
          n308 = Absolute Value(x=w483) -> (abs(x)=w482:dbl)
          n309 = Absolute Value(x=w481) -> (abs(x)=w480:dbl)
          n310 = Transpose 2D Array(2D array=w494) -> (transposed array=w493:dbl[][])
          n311 = Greater Or Equal?(x=w482, y=w480) -> (x >= y?=w485:bool)
          n312 = call "SaveDataFile.vi"("Arrays format"="%010.2f", "Humidity"=w490, "Array Titles"="Voltage[V] Current[nA]", "Temperature"=w491, "Actual array lengths"=w484, "no. of arrays"=2, "Data Array"=w493) -> ("Error Out"=w488:errorcluster, "Path + Filename OUT"=w508:string)  [unwired: 1 in, 2 out]
          n313 = call "WriteLogFile.vi"("Data File"=w508, "Error In"=w488, "DUT passed?"=w485, "Value TechSpec criteria"=w483, "Files saved?"=w489) -> ()  [unwired: 6 in, 1 out]
        }
      }
      n314 = Select(t="Run finished.\nData saved." ("STATUS 1"), s=w468, f="Run finished.\nData not saved." ("STATUS 1")) -> (s? t:f=w471:string)
      n315 = local write "STATUS 1"(w471) -> ()
      "Done!" <- w466
    }
  }
